vi "linx.vi"() -> ()   [LabVIEW 2020]
uses:
  <vilib>/MakerHub/LINX/Public/Peripherals/Analog/Analog Read 1 Chan.vi
  <vilib>/MakerHub/LINX/Public/Peripherals/Analog/Analog Read N Chans.vi
  <vilib>/MakerHub/LINX/Public/Peripherals/Digital/Digital Write N Chans.vi
  <vilib>/MakerHub/LINX/Private/Local IO/LinxAnalogRead.vi
  <vilib>/MakerHub/LINX/Public/Utilities/Check Channel.vi
  <vilib>/MakerHub/LINX/Private/Local IO/LinxDigitalWrite.vi
  <vilib>/MakerHub/LINX/Public/Utilities/Open Serial.vi
  <vilib>/MakerHub/LINX/Private/Utilties/Generate Error.vi
  <vilib>/MakerHub/LINX/Public/Peripherals/Digital/Digital Write 1 Chan.vi
  <vilib>/MakerHub/LINX/LMH-LINX.lvlib
panel:
  in  "Tab Control":enum32{"Page 1", "Page 2"}(tab)
  out "low water level":bool
  out "Raindrop":bool
  out "Loop Rate (Hz)":u32
  in  "stop":bool
  out "TDS Value (ppm)":dbl
  out "TDS Value Chart":dbl(graph)
  out "Raindrop value (mm)":dbl
  out "Water Level":dbl
  out "pump on/off":bool
  out "Water level":dbl(slide) scale=0.0..300.0
  out "raindrop value":dbl(slide) scale=0.0..200.0
  out "low TDS value":bool
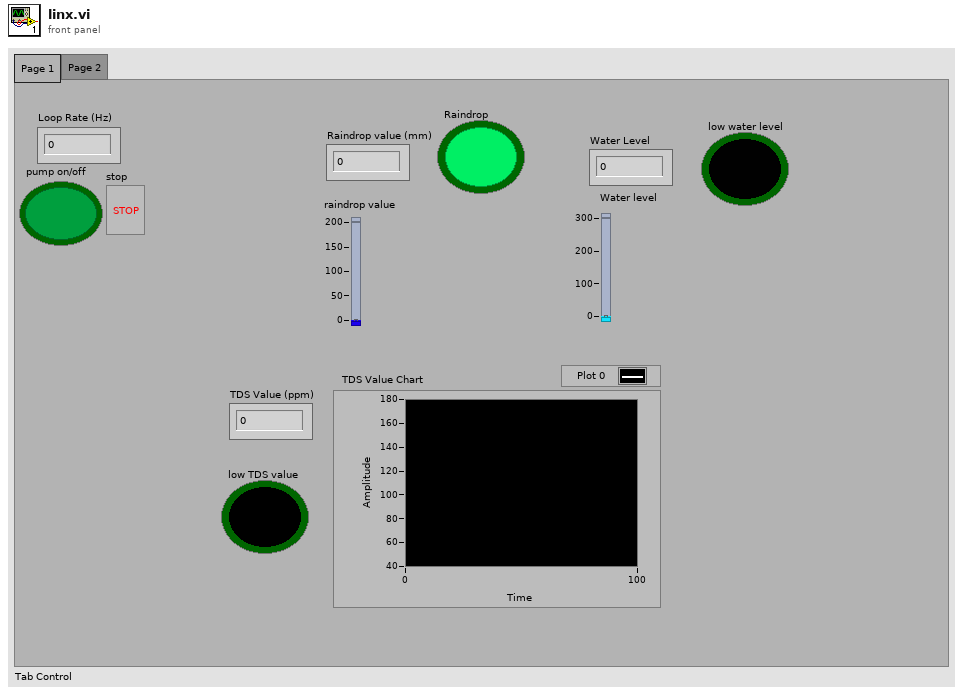
[diagram p1: front panel]
types:
  T1 = typedef "LMH-LINX.lvlib/LINX Ref.ctl" = cluster{"IO":T2, "Interface":T3, "LINX Device Config":T4}
  T2 = typedef "LMH-LINX.lvlib/Platform.ctl" = enum16{"Remote", "Local"}
  T3 = typedef "LMH-LINX.lvlib/Interface.ctl" = enum16{"Serial", "TCP"}
  T4 = typedef "LMH-LINX.lvlib/Device.lvlib/LINX Device Config.ctl" = cluster{"Interface":T3, "COM Port":refnum<visa-resource-name>, "TCP Configuration":T5, "Device Family":u8, "Device ID":u8, "Device Name":string, "TCP Ref":refnum<k5>, "Channels":T6}
  T5 = typedef "LMH-LINX.lvlib/Device.lvlib/TCP Config.ctl" = cluster{"IP Address":string, "Port":u16}
  T6 = typedef "LMH-LINX.lvlib/Channels.ctl" = cluster{"DI":u8[], "DO":u8[], "AI":u8[], "AO":u8[], "PWM":u8[], "QE":u8[], "UART":u8[], "I2C 2":u8[], "SPI":u8[], "CAN":u8[], "Servo":u8[], "AI Ref (V)":dbl, "AI Resolution (Bits)":u8, "AO Ref (V)":dbl, "AO Resolution (Bits)":u8}
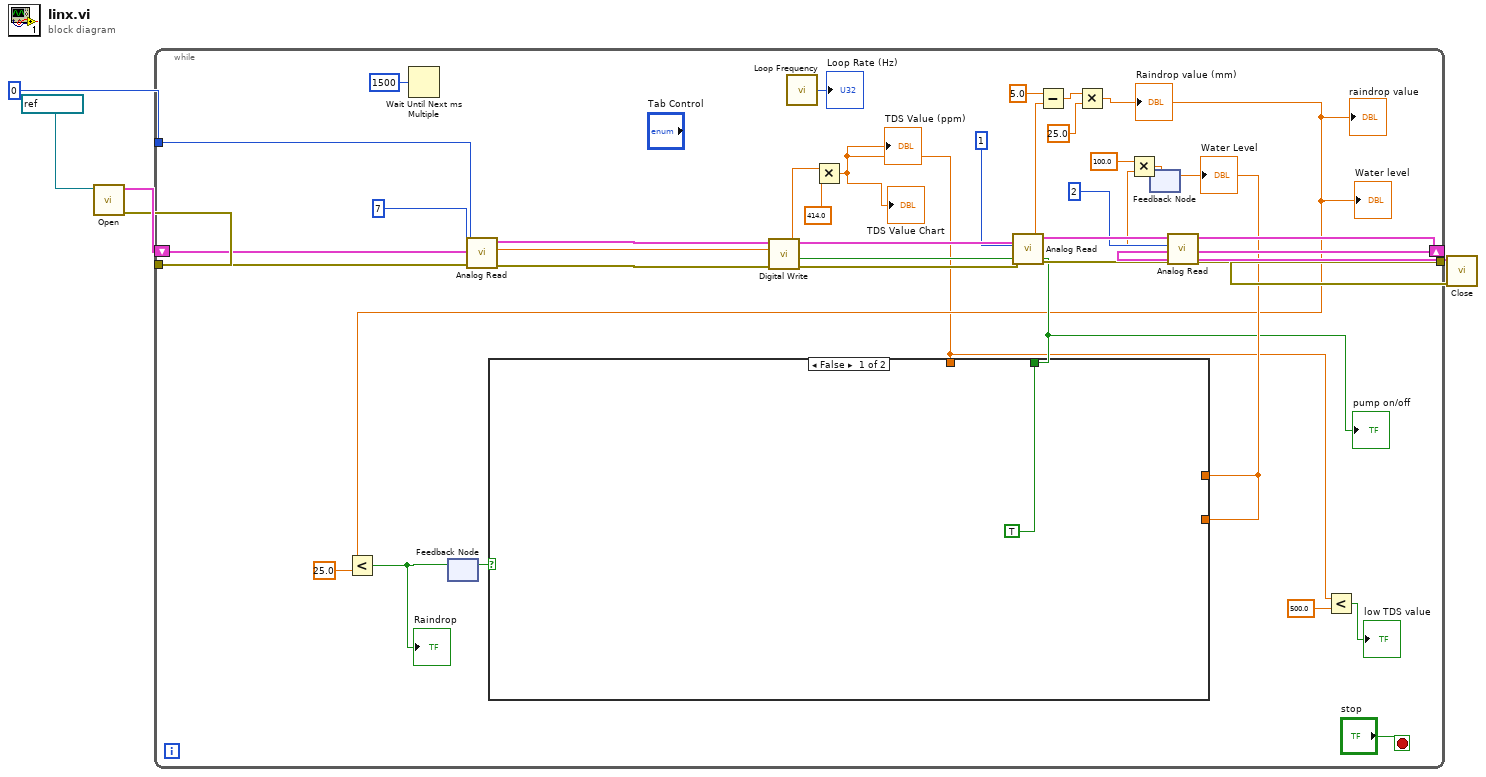
[diagram p0: block diagram]
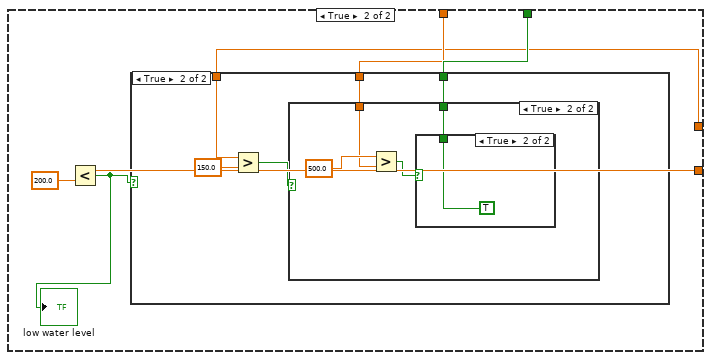
[diagram p2: hidden frame]
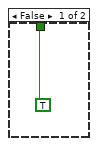
[diagram p3: hidden frame]
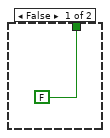
[diagram p4: hidden frame]
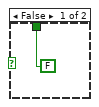
[diagram p5: hidden frame]
diagram:
  n1 = call-poly <vilib>:"Open.vi"("Serial Port"=refnum<visa-resource-name> "COM4") -> ("Error Out"=w2:errorcluster, "LINX Resource"=w6:T1)  [unwired: 8 in, 1 out]
  n2 = while {
    tunnel: u8 0 ("Analog Channel") -> [w40]
    shift-right: [w28] -> w5
    shift-left: w6 -> [w41]
    tunnel: w2 -> [w36]
    tunnel: [w25] -> w1
    stop <- "stop" stop-if-true
    n3 = Wait Until Next ms Multiple(millisecond multiple=u32 1500) -> ()  [unwired: 1 out]
    n4 = feedback #1() -> (w14:bool)  [unwired: 1 in]
    n5 = call-poly <vilib>:"Analog Read.vi"("Error In"=w36, "Analog Channel"=w40, "LINX Resource"=w41) -> ("Error Out"=w31:errorcluster, "Voltage"=w35:dbl, "LINX Resource"=w32:T1)  [unwired: 5 in, 1 out]
    n6 = call <vilib>:"Loop Frequency.vi"() -> ("Loop Rate (Hz)"=→"Loop Rate (Hz)":u32)
    n7 = Multiply(x=w35, y=414.0) -> (x*y=w9:dbl)
    "TDS Value (ppm)" <- w9
    "TDS Value Chart" <- w9
    n8 = feedback #2() -> (w13:dbl)  [unwired: 1 in]
    "Water Level" <- w13
    n9 = case shown="False" w14 {
      tunnel: [TRUE ("Output Value") w48] -> w12
      tunnel: w9 -> [_ w47]
      tunnel: w13 -> [_ w46]
      tunnel: w13 -> [_ w44]
      frame False {
      }
      frame True {
        n10 = Less?(x=w44, y=200.0) -> (x < y?=w43:bool)
        "low water level" <- w43
        n11 = case shown="True" w43 {
          tunnel: [TRUE ("Output Value") w54] -> w48
          tunnel: w47 -> [_ w53]
          tunnel: w46 -> [_ w51]
          frame False {
          }
          frame True {
            n12 = Greater?(x=w51, y=150.0) -> (0:w52:bool)
            n13 = case shown="True" w52 {
              tunnel: [FALSE ("Output Value") w59] -> w54
              tunnel: w53 -> [_ w57]
              frame False {
              }
              frame True {
                n14 = Greater?(x=500.0, y=w57) -> (0:w56:bool)
                n15 = case shown="True" w56 {
                  tunnel: [FALSE ("Output Value") TRUE ("Output Value")] -> w59
                  frame False {
                  }
                  frame True {
                  }
                }
              }
            }
          }
        }
      }
    }
    "pump on/off" <- w12
    n16 = call-poly <vilib>:"Digital Write.vi"("Error In"=w31, "Output Value"=w12, "DO Channel"=u8 7, "LINX Resource"=w32) -> ("Error Out"=w27:errorcluster, "LINX Resource"=w30:T1)  [unwired: 6 in]
    n17 = call-poly <vilib>:"Analog Read.vi"("Error In"=w27, "Analog Channel"=u8 1, "LINX Resource"=w30) -> ("Error Out"=w26:errorcluster, "Voltage"=w22:dbl, "LINX Resource"=w29:T1)  [unwired: 5 in, 1 out]
    n18 = Subtract(x=5.0, y=w22) -> (x-y=w20:dbl)
    n19 = Multiply(x=w20, y=25.0) -> (x*y=w11:dbl)
    "Raindrop value (mm)" <- w11
    "Water level" <- w11
    "raindrop value" <- w11
    n20 = Less?(x=w11, y=25.0) -> (x < y?=w10:bool)
    "Raindrop" <- w10
    n21 = feedback-in #1(w10) -> ()
    n22 = call-poly <vilib>:"Analog Read.vi"("Error In"=w26, "Analog Channel"=u8 2, "LINX Resource"=w29) -> ("Error Out"=w25:errorcluster, "Voltage"=w18:dbl, "LINX Resource"=w28:T1)  [unwired: 5 in, 1 out]
    n23 = Multiply(x=100.0, y=w18) -> (x*y=w16:dbl)
    n24 = feedback-in #2(w16) -> ()
    n25 = Less?(x=w9, y=500.0) -> (x < y?=→"low TDS value":bool)
  }
  n26 = call <vilib>:"Close.vi"("Error In"=w1, "LINX Resource"=w5) -> ()  [unwired: 9 in, 1 out]
